vi "Write--init.vi"(8 "error in (no error)":errorcluster, 10 "Motor params":T1={"Tipo"=0, "Dirección"=0, "N°. Pasos"=200, "Frecuencia (Hz)"=255, "Tipo de paso"=1} caption="Parámetros del motor" {"Tipo de paso" items=["Medio paso", "Paso completo"]; "Dirección" items=["Izquierda", "Derecha"]; "Tipo" items=["Unipolar", "Bipolar"]}, 11 "VISA resource name":refnum<visa-resource-name>) -> (0 "error out":errorcluster, 2 "Comando(string)":string, 3 "VISA resource name out":refnum<visa-resource-name>)   [LabVIEW 2020, in "Control de MaP.lvlib"]
doc: "convierte la selección de comando a cadena y lo envía al puerto seleccionado"
uses:
  Control de MaP.lvlib
  Controls/Command to motor.ctl
  <vilib>/Instr/_visa.llb/VISA Flush IO Buffer Mask.ctl
panel:
  out "return count":u32
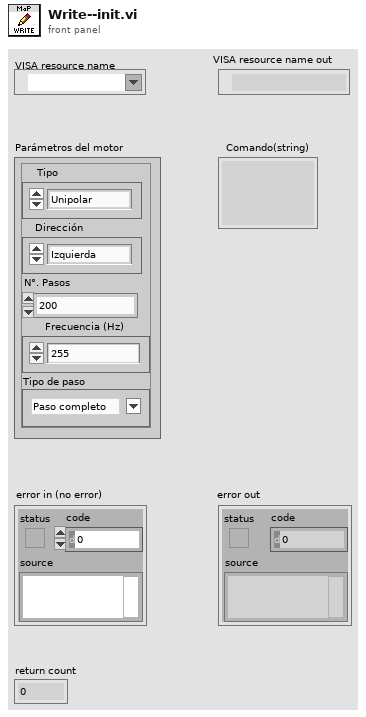
[diagram p1: front panel]
types:
  T1 = typedef "Control de MaP.lvlib/Command to motor.ctl" = cluster{"Tipo":u8, "Dirección":u8, "N°. Pasos":u16, "Frecuencia (Hz)":u8, "Tipo de paso":u8}
  T2 = typedef "VISA Flush IO Buffer Mask.ctl" = u16
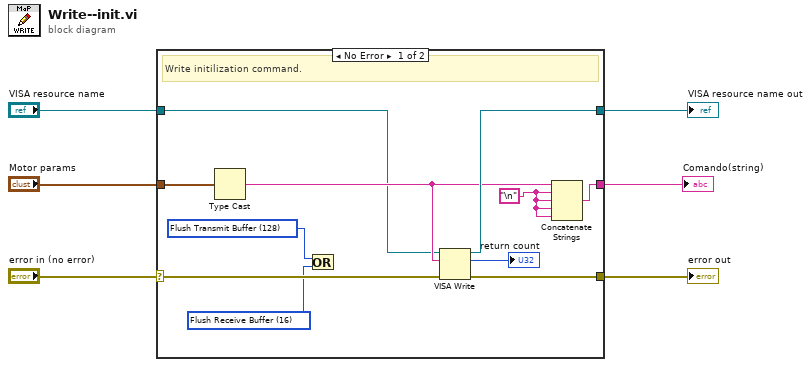
[diagram p0: block diagram]
diagram:
  n1 = case shown="No Error" "error in (no error)" {
    selector: "error in (no error)" -> [w11 w19]
    tunnel: [w13 _] -> w6
    tunnel: "VISA resource name" -> [w10 w18]
    tunnel: [w17 w18] -> w4
    tunnel: [w16 w19] -> w2
    tunnel: "Motor params" -> [w15 _]
    frame No Error {
      w7 = "\n"
      w8 = T2 16 items=["Flush Receive Buffer"=16, "Write Transmit Buffer to Device"=32, "Flush Receive Buffer (No I/O)"=64, "Flush Transmit Buffer"=128] ("y")
      w9 = T2 128 items=["Flush Receive Buffer"=16, "Write Transmit Buffer to Device"=32, "Flush Receive Buffer (No I/O)"=64, "Flush Transmit Buffer"=128] ("Mask")
      # "Write initilization command."
      n2 = Type Cast(x=w15) -> (*(type *) &x=w14:string)  [unwired: 1 in]
      n3 = Or(x=w9, y=w8) -> ()  [unwired: 1 out]
      n4 = VISA Write(VISA resource name=w10, write buffer=w14, error in (no error)=w11) -> (VISA resource name out=w17:refnum<visa-resource-name>, return count=→"return count":u32, error out=w16:errorcluster)
      n5 = Concatenate Strings(w14, w7, w7, w7, w7) -> (w13:string)
    }
    frame Error {
    }
  }
  "VISA resource name out" <- w4
  "error out" <- w2
  "Comando(string)" <- w6
